vi "Set Attr Dict.vi"(7 "Tree ID":string, 8 "Error In":errorcluster, 10 "Attributes Dictionary":variant, 11 "Tree Manager":T1) -> (0 "Error Out":errorcluster, 3 "Tree Manager":T1)   [LabVIEW 2016, in "Tree Manager.lvclass"]
doc: "Set input variant as the attribute dictionary for the Tree. \n\n<b>WARNING</b> This removes any previous attributes."
uses:
  Tree Manager.lvclass
  Typedefs/Session Handle.ctl
  Tree Manager.lvclass/Tree Manager.ctl
  Typedefs/Tree.ctl
  <vilib>/Utility/error.llb/Error Cluster From Error Code.vi
  <vilib>/ErrorRing/Error Ring.xnode
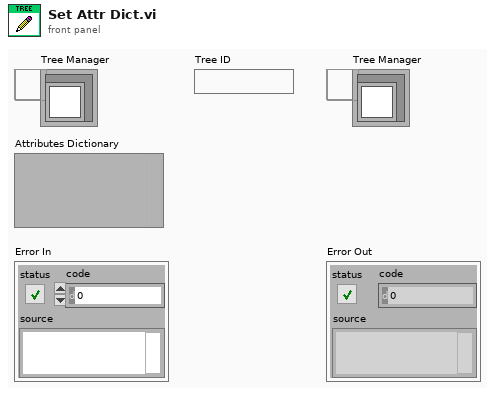
[diagram p1: front panel]
types:
  T1 = typedef "Tree Manager.lvclass/Session Handle.ctl" = refnum<data-value>
  T2 = typedef "Tree Manager.lvclass/Tree.ctl" = cluster{"Unique ID":string, "Parent ID":string, "Child IDs":string[], "Data":variant, "Name":string}
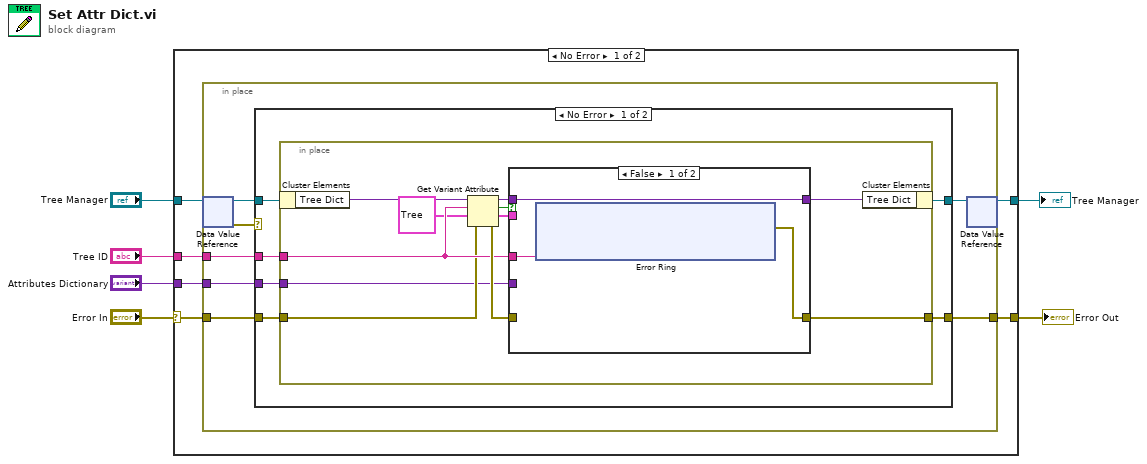
[diagram p0: block diagram]
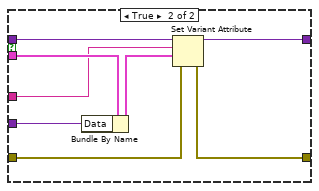
[diagram p2: hidden frame]
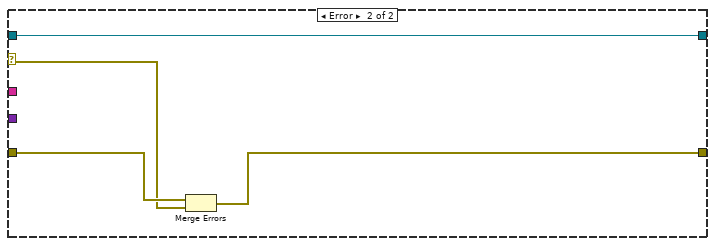
[diagram p3: hidden frame]
diagram:
  n1 = case shown="No Error" "Error In" {
    selector: "Error In" -> [w10 w59]
    tunnel: "Tree Manager" -> [w12 w60]
    tunnel: [w11 w60] -> w5
    tunnel: [w9 w59] -> w3
    tunnel: "Tree ID" -> [w8 _]
    tunnel: "Attributes Dictionary" -> [w7 _]
    frame No Error {
      n2 = in-place {
        in-place-border: w10 -> [w15]
        in-place-border: [w18] -> w9
        in-place-border: w8 -> [w14]
        in-place-border: w7 -> [w13]
        n3 = in-place-dvr #1(w12) -> (w19:refnum<class "Tree Manager.lvclass">, w16:errorcluster)
        n4 = case shown="No Error" w16 {
          selector: w16 -> [_ w57]
          tunnel: w19 -> [w25 w55]
          tunnel: [w24 w56] -> w18
          tunnel: [w23 w55] -> w17
          tunnel: w15 -> [w22 w58]
          tunnel: w14 -> [w21 _]
          tunnel: w13 -> [w20 _]
          frame No Error {
            n5 = in-place {
              in-place-border: [w28] -> w24
              in-place-border: w22 -> [w29]
              in-place-border: w21 -> [w30]
              in-place-border: w20 -> [w26]
              n6 = in-place-cluster #2(w25) -> ("Tree Dict"=w32:variant)
              n7 = Get Variant Attribute(Variant=w32, name=w30, default value (empty Variant)=T2 {"Unique ID"="", "Parent ID"="", "Child IDs"=[], "Data"=variant, "Name"=""} ("Cluster of class private data"), error in=w29) -> (duplicate Variant=w35:variant, found=w33:bool, value=w34:T2, error out=w36:errorcluster)
              n8 = case shown="False" w33 {
                tunnel: w34 -> [_ w50]
                tunnel: w35 -> [w39 w54]
                tunnel: w36 -> [_ w51]
                tunnel: [w38 w52] -> w28
                tunnel: [w39 w53] -> w31
                tunnel: w30 -> [w37 w48]
                tunnel: w26 -> [_ w47]
                frame False {
                  n9 = xnode "Error Ring"("parameter 0"=w37) -> ("error out"=w38:errorcluster)
                }
                frame True {
                  n10 = Bundle By Name(cluster=w50, "Data"=w47) -> (w49:T2)
                  n11 = Set Variant Attribute(Variant=w54, name=w48, value=w49, error in=w51) -> (Variant out=w53:variant, error out=w52:errorcluster)  [unwired: 1 out]
                }
              }
              n12 = in-place-cluster #2("Tree Dict"=w31) -> (w23:refnum<class "Tree Manager.lvclass">)
            }
          }
          frame Error {
            n13 = Merge Errors(w58, w57) -> (w56:errorcluster)
          }
        }
        n14 = in-place-dvr #1(w17) -> (w11:T1)  [unwired: 1 out]
      }
    }
    frame Error {
    }
  }
  "Tree Manager" <- w5
  "Error Out" <- w3
